vi "LCR_Readout.vi"(8 "error in (no error)":errorcluster, 11 "LCRControl in":refnum<class "LCRControl.lvclass">) -> (0 "error out":errorcluster, 1 "Resistance in Ohm":dbl, 2 "Capacitance in pF":dbl, 3 "LCRControl out":refnum<class "LCRControl.lvclass">)   [LabVIEW 2018, in "LCRControl.lvclass"]
uses:
  LCRControl.lvclass
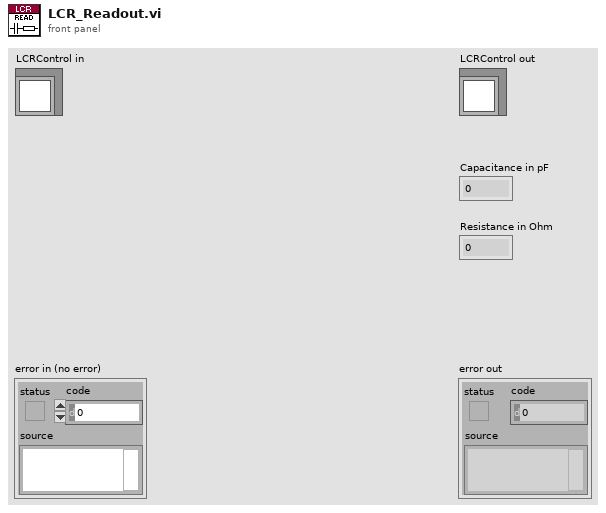
[diagram p1: front panel]
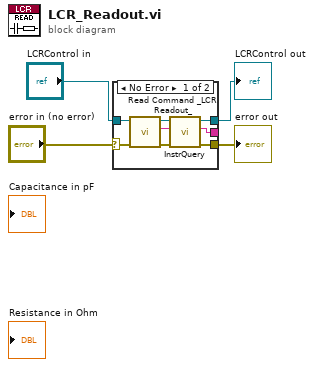
[diagram p0: block diagram]
diagram:
  n1 = case shown="No Error" "error in (no error)" {
    selector: "error in (no error)" -> [w8 w14]
    tunnel: [w7 w14] -> w3
    tunnel: [w12 w13] -> w1
    tunnel: "LCRControl in" -> [w6 w13]
    tunnel: [w5 _] -> _
    frame No Error {
      n2 = call-dynamic "Read Command _LCR Readout_.vi"("error in (no error)"=w8, "LCRControl in"=w6) -> ("error out"=w9:errorcluster, "Command \"LCR Readout\""=w10:string, "LCRControl out"=w11:refnum<class "LCRControl.lvclass">)  [unwired: 7 in]
      n3 = call-dynamic "InstrQuery.vi"("error in (no error)"=w9, "Command string"=w10, "InstControl in"=w11) -> ("error out"=w7:errorcluster, "Instrument response"=w5:string, "InstControl out"=w12:refnum<class "LCRControl.lvclass">)  [unwired: 6 in]
    }
    frame Error {
    }
  }
  "error out" <- w3
  "LCRControl out" <- w1
